vi "Rhythm-Initialize.vi"(0 "Rhythm":T2={"Method"=enum."Telegraph", "Waveform"=enum."Click", "Time"={"Ramp (ms)"=1.0, "Duration (ms)"=2.0, "Interval (ms)"=1.0}, "Expr"="", "Pattern"={"# rand"=0.0, "reg fraction"=0.0, "Rcyc"=0, "pattern"=enum."RAND-REG", "Lsignal (cyc)"={"Min"=0, "Max"=0}, "Trans (cyc)"={"Min"=0, "Max"=0}}} caption="ToneCloud", 7 "Sampling rate (Hz)":dbl=50000.0, 9 "Npts":i32, 11 "error in (no error)":errorcluster) -> (3 "#frames":i32, 4 "Values":dbl[](array[numeric]), 6 "Mask":i32[](array[numeric]), 8 "Data":T1, 15 "error out":errorcluster)   [LabVIEW 2020]
uses:
  Rhythm-Properties.ctl
  Rhythm-Data.ctl
  Rhythm-Initialization Action.ctl
  Utility VIs/Math VIs/LinSpace (x0-dx-npts).vi
  Utility VIs/Array Manipulation VIs/Irregular Array Subset (I32).vi
  <vilib>/Analysis/1siggen.llb/Riffle Array (I32).vi
  <vilib>/Analysis/NI_AALBase.lvlib
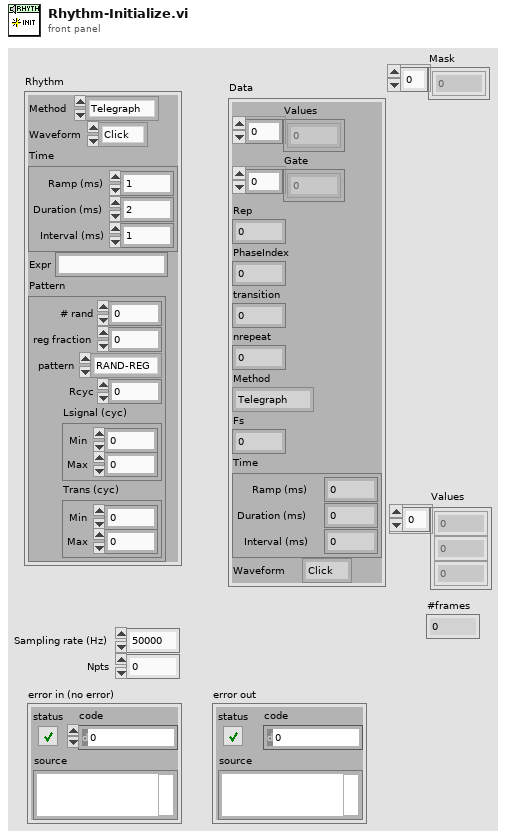
[diagram p1: front panel]
types:
  T1 = typedef "Rhythm-Data.ctl" = cluster{"Values":dbl[], "Gate":dbl[], "Rep":i32, "PhaseIndex":i32, "transition":i32, "nrepeat":i32, "Method":enum16{"Telegraph", "Interval"}, "Fs":dbl, "Time":cluster{"Ramp (ms)":dbl, "Duration (ms)":dbl, "Interval (ms)":dbl}, "Waveform":enum16{"Click", "Noise"}}
  T2 = typedef "Rhythm-Properties.ctl" = cluster{"Method":enum16{"Telegraph", "Interval"}, "Waveform":enum16{"Click", "Noise"}, "Time":cluster{"Ramp (ms)":dbl, "Duration (ms)":dbl, "Interval (ms)":dbl}, "Expr":string, "Pattern":cluster{"# rand":dbl, "reg fraction":dbl, "Rcyc":i32, "pattern":enum16{"RAND-REG", "REG-RAND", "RAND", "REG", "STEP", "CF"}, "Lsignal (cyc)":cluster{"Min":i32, "Max":i32}, "Trans (cyc)":cluster{"Min":i32, "Max":i32}}}
  T3 = typedef "Rhythm-Initialization Action.ctl" = enum16{"Start", "Rand", "Reg", "Titrate", "Signal", "Done"}
  T4 = cluster{"Duration (ms)":dbl, "Interval (ms)":dbl, "Ramp (ms)":dbl}
  T5 = cluster{"Ramp (ms)":dbl, "Duration (ms)":dbl, "Interval (ms)":dbl}
  T6 = enum16{"RAND-REG", "REG-RAND", "RAND", "REG", "STEP", "CF"}
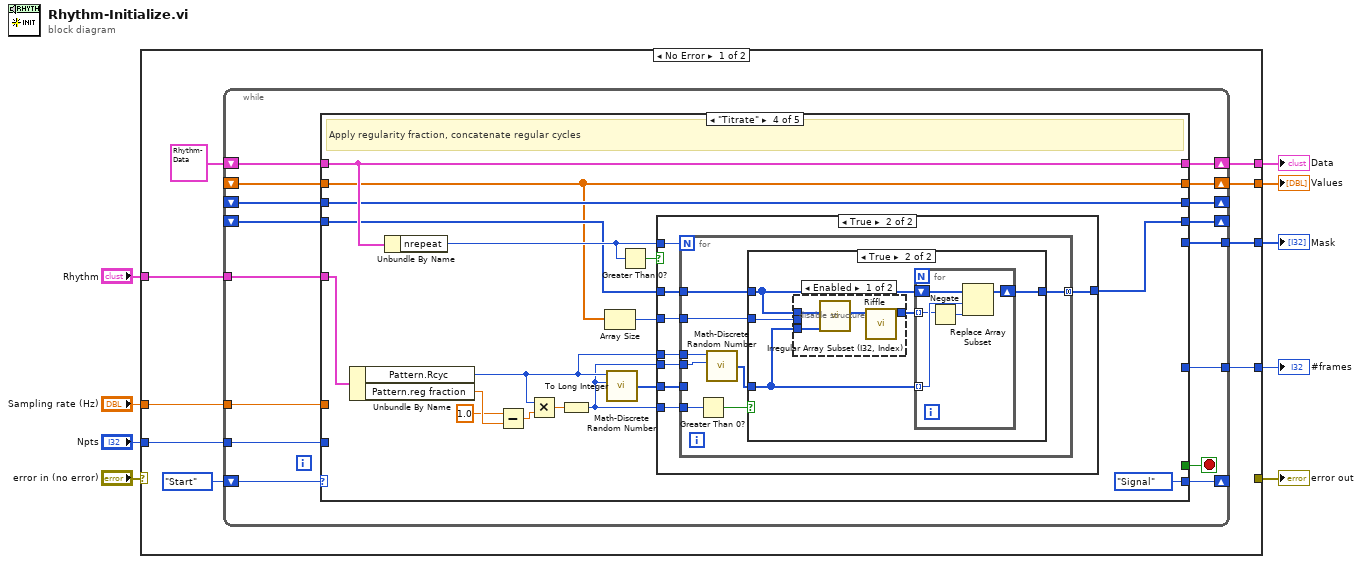
[diagram p0: block diagram]
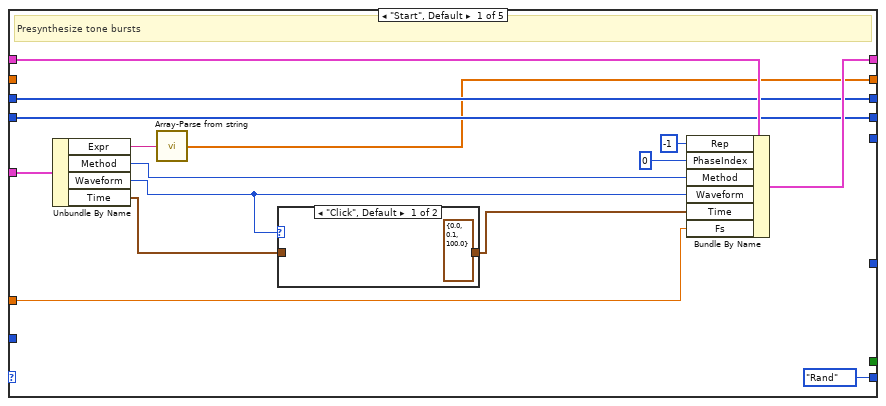
[diagram p2: hidden frame]
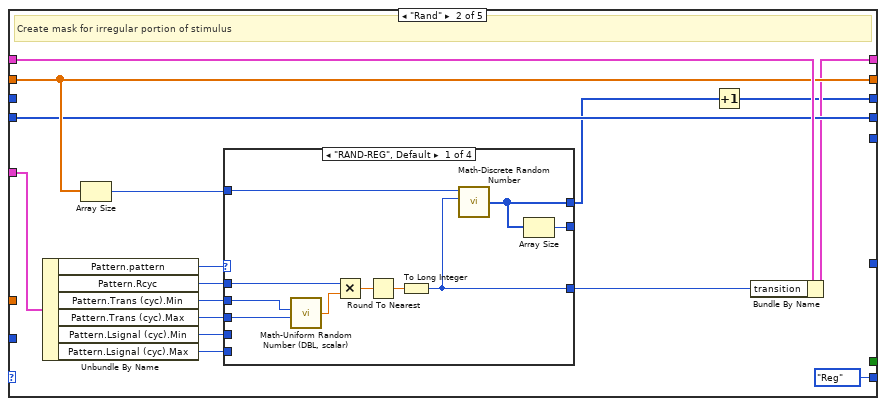
[diagram p4: hidden frame]
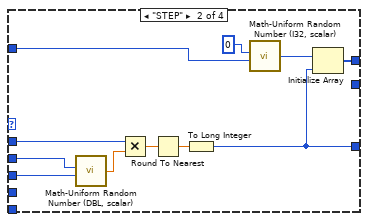
[diagram p5: hidden frame]
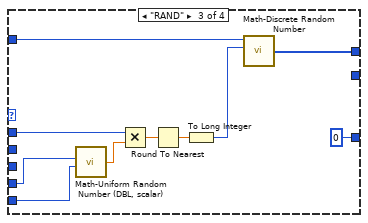
[diagram p6: hidden frame]
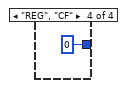
[diagram p7: hidden frame]
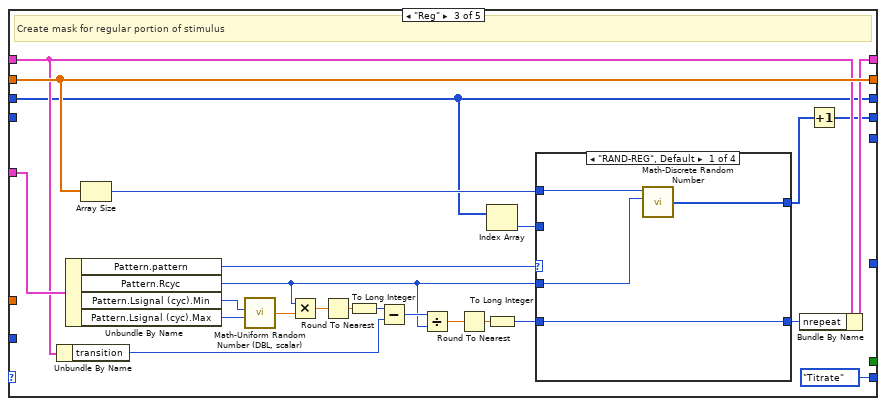
[diagram p8: hidden frame]
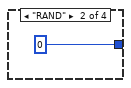
[diagram p9: hidden frame]
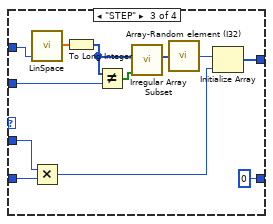
[diagram p10: hidden frame]
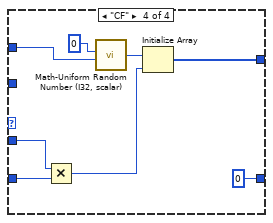
[diagram p11: hidden frame]
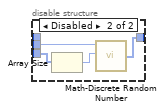
[diagram p14: hidden frame]
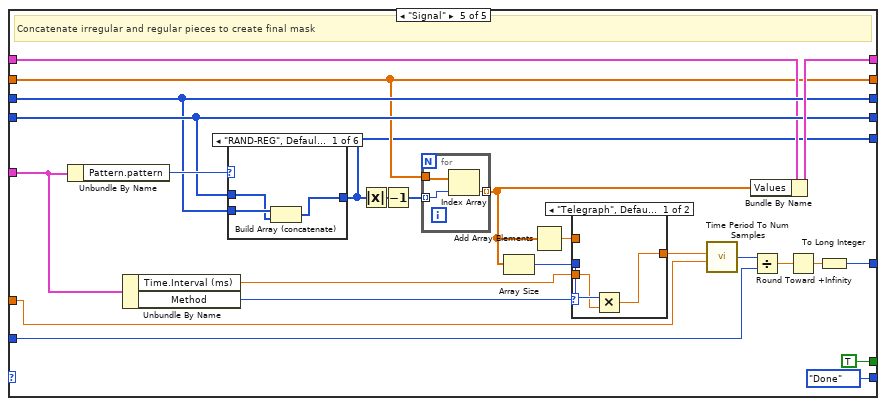
[diagram p15: hidden frame]
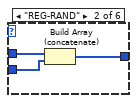
[diagram p17: hidden frame]
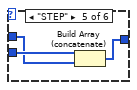
[diagram p20: hidden frame]
diagram:
  n1 = case shown="No Error" "error in (no error)" {
    selector: "error in (no error)" -> [_ w245]
    tunnel: [_ w245] -> w6
    tunnel: "Sampling rate (Hz)" -> [w17 _]
    tunnel: "Npts" -> [w13 _]
    tunnel: "Rhythm" -> [w16 _]
    tunnel: [w18 _] -> w4
    tunnel: [w14 _] -> w3
    tunnel: [w12 _] -> w2
    tunnel: [w10 _] -> w1
    frame No Error {
      n2 = while {
        tunnel: w17 -> [w33]
        tunnel: w16 -> [w32]
        shift-right: [w34] -> w18
        shift-left: T1 {"Values"=[], "Gate"=[], "Rep"=0, "PhaseIndex"=0, "transition"=0, "nrepeat"=0, "Method"=enum."Telegraph", "Fs"=0.0, "Time"={"Ramp (ms)"=0.0, "Duration (ms)"=0.0, "Interval (ms)"=0.0}, "Waveform"=enum."Click"} ("Data") -> [w31]
        shift-right: [w30] -> _
        shift-left: _ -> [w29]
        shift-right: [w28] -> w14
        shift-left: _ -> [w27]
        shift-right: [w26] -> _
        shift-left: _ -> [w25]
        tunnel: w13 -> [w23]
        tunnel: [w22] -> w12
        shift-right: [w20] -> _
        shift-left: Rhythm-Initialization_Action."Start" -> [w21]
        tunnel: [w19] -> w10
        stop <- w24 stop-if-true
        n3 = case shown="\"Titrate\"" w21 {
          tunnel: [w49 w59 w108 w165 w225] -> w34
          tunnel: w33 -> [w39 _ _ _ w208]
          tunnel: w32 -> [w48 w67 w123 w164 w214]
          tunnel: w31 -> [w47 w66 w114 w165 w220]
          tunnel: [w46 w52 w104 w162 w222] -> w30
          tunnel: w29 -> [w46 _ w104 w162 w222]
          tunnel: [w43 w65 w122 w153 w213] -> w28
          tunnel: w27 -> [_ w65 w122 w153 w213]
          tunnel: [w45 w64 w100 w160 w223] -> w26
          tunnel: w25 -> [w45 w64 _ w154 w223]
          tunnel: [_ _ _ _ TRUE] -> w24
          tunnel: w23 -> [_ _ _ _ w219]
          tunnel: [_ _ _ _ w216] -> w22
          tunnel: [Rhythm-Initialization_Action."Rand" Rhythm-Initialization_Action."Reg" Rhythm-Initialization_Action."Titrate" Rhythm-Initialization_Action."Signal" Rhythm-Initialization_Action."Done"] -> w20
          tunnel: [_ _ _ _ w202] -> w19
          frame "Start", Default {
            # "Presynthesize tone bursts"
            n4 = Unbundle By Name(w48) -> ("Expr"=w44:string, "Method"=w41:enum16{"Telegraph", "Interval"}, "Waveform"=w38:enum16{"Click", "Noise"}, "Time"=w37:T5)
            n5 = call "Array-Parse from string.vi"("String"=w44) -> ("Array"=w43:dbl[])  [unwired: 13 in, 1 out]
            n6 = case shown="\"Click\", Default" w38 {
              tunnel: w37 -> [_ w51]
              tunnel: [T4 {"Duration (ms)"=0.0, "Interval (ms)"=0.1, "Ramp (ms)"=100.0} ("Time") w51] -> w36
              frame "Click", Default {
              }
              frame "Noise" {
              }
            }
            n7 = Bundle By Name(cluster=w47, "Rep"=-1, "PhaseIndex"=0 ("Index"), "Method"=w41, "Waveform"=w38, "Time"=w36, "Fs"=w39) -> (w49:T1)
          }
          frame "Rand" {
            # "Create mask for irregular portion of stimulus"
            n8 = Unbundle By Name(w67) -> ("Pattern.pattern"=w57:T6, "Pattern.Rcyc"=w61:i32, "Pattern.Trans (cyc).Min"=w63:i32, "Pattern.Trans (cyc).Max"=w62:i32, "Pattern.Lsignal (cyc).Min"=w56:i32, "Pattern.Lsignal (cyc).Max"=w55:i32)
            n9 = Array Size(array=w65) -> (size(s)=w60:i32)
            n10 = case shown="\"RAND-REG\", Default" w57 {
              tunnel: w63 -> [w77 w88 _ _]
              tunnel: w62 -> [w76 w87 _ _]
              tunnel: w61 -> [w75 w86 w98 _]
              tunnel: w60 -> [w74 w82 w97 _]
              tunnel: [w69 w79 w96 _] -> w54
              tunnel: [w70 w78 0 0] -> w58
              tunnel: w56 -> [_ _ w91 _]
              tunnel: w55 -> [_ _ w90 _]
              tunnel: [w68 _ _ _] -> _
              frame "RAND-REG", Default {
                n11 = call "Math-Uniform Random Number (DBL, scalar).vi"("Ymax"=w76, "Ymin"=w77) -> ("Random Value"=w73:dbl)  [unwired: 4 in]
                n12 = Multiply(x=w75, y=w73) -> (x*y=w72:dbl)
                n13 = Round To Nearest(number=w72) -> (nearest integer value=w71:dbl)
                n14 = To Long Integer(number=w71) -> (32bit integer=w70:i32)
                n15 = call "Math-Discrete Random Number.vi"("N"=w70, "samples"=w74) -> ("Random Values"=w69:i32[])  [unwired: 4 in]
                n16 = Array Size(array=w69) -> (size(s)=w68:i32)
              }
              frame "STEP" {
                n17 = call "Math-Uniform Random Number (DBL, scalar).vi"("Ymax"=w87, "Ymin"=w88) -> ("Random Value"=w85:dbl)  [unwired: 4 in]
                n18 = Multiply(x=w86, y=w85) -> (x*y=w84:dbl)
                n19 = Round To Nearest(number=w84) -> (nearest integer value=w83:dbl)
                n20 = To Long Integer(number=w83) -> (32bit integer=w78:i32)
                n21 = call "Math-Uniform Random Number (I32, scalar).vi"("Ymax"=w82, "Ymin"=0) -> ("Random Int"=w80:i32)  [unwired: 4 in]
                n22 = Initialize Array(w80, w78) -> (w79:i32[])
              }
              frame "RAND" {
                n23 = call "Math-Uniform Random Number (DBL, scalar).vi"("Ymax"=w90, "Ymin"=w91) -> ("Random Value"=w95:dbl)  [unwired: 4 in]
                n24 = Multiply(x=w98, y=w95) -> (x*y=w94:dbl)
                n25 = Round To Nearest(number=w94) -> (nearest integer value=w93:dbl)
                n26 = To Long Integer(number=w93) -> (32bit integer=w92:i32)
                n27 = call "Math-Discrete Random Number.vi"("N"=w92, "samples"=w97) -> ("Random Values"=w96:i32[])  [unwired: 4 in]
              }
              frame "REG", "CF" {
              }
            }
            n28 = Increment(x=w54) -> (x+1=w52:i32[])
            n29 = Bundle By Name(cluster=w66, "transition"=w58) -> (w59:T1)
          }
          frame "Reg" {
            # "Create mask for regular portion of stimulus"
            n30 = Unbundle By Name(w114) -> ("transition"=w112:i32)
            n31 = Unbundle By Name(w123) -> ("Pattern.pattern"=w106:T6, "Pattern.Rcyc"=w105:i32, "Pattern.Lsignal (cyc).Min"=w116:i32, "Pattern.Lsignal (cyc).Max"=w115:i32)
            n32 = Array Size(array=w122) -> (size(s)=w121:i32)
            n33 = call "Math-Uniform Random Number (DBL, scalar).vi"("Ymax"=w115, "Ymin"=w116) -> ("Random Value"=w117:dbl)  [unwired: 4 in]
            n34 = Multiply(x=w105, y=w117) -> (x*y=w118:dbl)
            n35 = Round To Nearest(number=w118) -> (nearest integer value=w119:dbl)
            n36 = To Long Integer(number=w119) -> (32bit integer=w113:i32)
            n37 = Subtract(x=w113, y=w112) -> (x-y=w111:i32)
            n38 = Divide(x=w111, y=w105) -> (x/y=w110:dbl)
            n39 = Round To Nearest(number=w110) -> (nearest integer value=w109:dbl)
            n40 = Index Array(array=w104) -> (element=w103:i32)  [unwired: 1 in]
            n41 = To Long Integer(number=w109) -> (32bit integer=w101:i32)
            n42 = case shown="\"RAND-REG\", Default" w106 {
              tunnel: w121 -> [w127 _ w133 w145]
              tunnel: [w126 _ w135 w141] -> w120
              tunnel: [w124 0 0 0] -> w107
              tunnel: w101 -> [w124 _ w138 w144]
              tunnel: w105 -> [w125 _ w137 w143]
              tunnel: w103 -> [_ _ w140 _]
              frame "RAND-REG", Default {
                n43 = call "Math-Discrete Random Number.vi"("N"=w125, "samples"=w127) -> ("Random Values"=w126:i32[])  [unwired: 4 in]
              }
              frame "RAND" {
              }
              frame "STEP" {
                n44 = call-poly "LinSpace.vi"("npts"=w133) -> ("Array"=w132:dbl[])  [unwired: 3 in, 1 out]
                n45 = Multiply(x=w137, y=w138) -> (x*y=w136:i32)
                n46 = To Long Integer(number=w132) -> (32bit integer=w130:i32[])
                n47 = Not Equal?(x=w130, y=w140) -> (x != y?=w131:bool[])
                n48 = call-poly "Irregular Array Subset.vi"("Mask"=w131, "Array"=w130) -> ("Array Subset"=w129:i32[])  [unwired: 8 in, 1 out]
                n49 = call "Array-Random element (I32).vi"("Array"=w129) -> ("Element"=w134:i32)  [unwired: 1 in, 1 out]
                n50 = Initialize Array(w134, w136) -> (w135:i32[])
              }
              frame "CF" {
                n51 = Multiply(x=w143, y=w144) -> (x*y=w142:i32)
                n52 = call "Math-Uniform Random Number (I32, scalar).vi"("Ymax"=w145, "Ymin"=0) -> ("Random Int"=w146:i32)  [unwired: 4 in]
                n53 = Initialize Array(w146, w142) -> (w141:i32[])
              }
            }
            n54 = Bundle By Name(cluster=w114, "nrepeat"=w107) -> (w108:T1)
            n55 = Increment(x=w120) -> (x+1=w100:i32[])
          }
          frame "Titrate" {
            # "Apply regularity fraction, concatenate regular cycles"
            n56 = Unbundle By Name(w164) -> ("Pattern.Rcyc"=w151:i32, "Pattern.reg fraction"=w156:dbl)
            n57 = Unbundle By Name(w165) -> ("nrepeat"=w159:i32)
            n58 = Subtract(x=1.0, y=w156) -> (x-y=w157:dbl)
            n59 = Multiply(x=w151, y=w157) -> (x*y=w163:dbl)
            n60 = To Long Integer(number=w163) -> (32bit integer=w150:i32)
            n61 = Array Size(array=w153) -> (size(s)=w152:i32)
            n62 = call "Math-Discrete Random Number.vi"("N"=w150, "samples"=w151) -> ("Random Values"=w161:i32[])  [unwired: 4 in]
            n63 = Greater Than 0?(x=w159) -> (x > 0?=w158:bool)
            n64 = case shown="True" w158 {
              tunnel: w159 -> [_ w174]
              tunnel: w154 -> [w166 w173]
              tunnel: w161 -> [_ w172]
              tunnel: w150 -> [_ w171]
              tunnel: [w166 w170] -> w160
              tunnel: w152 -> [_ w169]
              tunnel: w151 -> [_ w168]
              tunnel: w150 -> [_ w167]
              frame False {
              }
              frame True {
                n65 = for {
                  N: w174 -> [_]
                  tunnel: w173 -> [w180]
                  tunnel: w172 -> [_]
                  tunnel: w171 -> [w182]
                  tunnel: [w179] -> w170 mode=concatenating
                  tunnel: w169 -> [w178]
                  tunnel: w168 -> [w177]
                  tunnel: w167 -> [w176]
                  n66 = Greater Than 0?(x=w182) -> (x > 0?=w181:bool)
                  n67 = call "Math-Discrete Random Number.vi"("N"=w176, "samples"=w177) -> ("Random Values"=w175:i32[])  [unwired: 4 in]
                  n68 = case shown="True" w181 {
                    tunnel: w180 -> [w183 w188]
                    tunnel: w175 -> [_ w185]
                    tunnel: [w183 w187] -> w179
                    tunnel: w178 -> [_ w184]
                    frame False {
                    }
                    frame True {
                      n69 = disable-structure shown="Enabled" {
                        disable-tunnel: w188 -> [w191 _]
                        disable-tunnel: [w190 w193] -> w186
                        disable-tunnel: w185 -> [w189 w196]
                        disable-tunnel: w184 -> [_ w195]
                        frame Enabled {
                          n70 = call "Irregular Array Subset (I32, Index).vi"("Indices"=w189, "Array"=w191) -> ("Array Subset"=w192:i32[])  [unwired: 8 in, 1 out]
                          n71 = call-poly <vilib>:"Riffle.vi"("X"=w192) -> ("Riffled {X}"=w190:i32[])  [unwired: 8 in, 2 out]
                        }
                        frame Disabled {
                          n72 = Array Size(array=w196) -> (size(s)=w194:i32)
                          n73 = call "Math-Discrete Random Number.vi"("N"=w194, "samples"=w195) -> ("Random Values"=w193:i32[])  [unwired: 4 in]
                        }
                      }
                      n74 = for {
                        shift-right: [w200] -> w187
                        shift-left: w188 -> [w201]
                        tunnel: w186 -> [w198] mode=indexing
                        tunnel: w185 -> [w199] mode=indexing
                        n75 = Negate(x=w198) -> (-x=w197:i32)
                        n76 = Replace Array Subset(array=w201, new element=w197, index=w199) -> (w200:i32[])
                      }
                    }
                  }
                }
              }
            }
          }
          frame "Signal" {
            # "Concatenate irregular and regular pieces to create final mask"
            n77 = Unbundle By Name(w214) -> ("Pattern.pattern"=w224:T6)
            n78 = Unbundle By Name(w214) -> ("Time.Interval (ms)"=w205:dbl, "Method"=w212:enum16{"Telegraph", "Interval"})
            n79 = case shown="\"RAND-REG\", Default" w224 {
              tunnel: w223 -> [w234 w238 _ w240 w242 _]
              tunnel: w222 -> [w235 w237 w239 _ w243 w244]
              tunnel: [w233 w236 w239 w240 w241 w244] -> w202
              frame "RAND-REG", Default {
                n80 = Build Array (concatenate)(w235, w234) -> (w233:i32[])
              }
              frame "REG-RAND" {
                n81 = Build Array (concatenate)(w238, w237) -> (w236:i32[])
              }
              frame "RAND" {
              }
              frame "REG" {
              }
              frame "STEP" {
                n82 = Build Array (concatenate)(w243, w242) -> (w241:i32[])
              }
              frame "CF" {
              }
            }
            n83 = Absolute Value(x=w202) -> (abs(x)=w204:i32[])
            n84 = Decrement(x=w204) -> (x-1=w203:i32[])
            n85 = for {
              tunnel: w213 -> [w232]
              tunnel: w203 -> [w231] mode=indexing
              tunnel: [w230] -> w206 mode=indexing
              n86 = Index Array(array=w232, index=w231) -> (element=w230:dbl)
            }
            n87 = Array Size(array=w206) -> (size(s)=w207:i32)
            n88 = Add Array Elements(numeric array=w206) -> (sum=w211:dbl)
            n89 = case shown="\"Telegraph\", Default" w212 {
              tunnel: w207 -> [w228 _]
              tunnel: w205 -> [w227 _]
              tunnel: [w226 w229] -> w209
              tunnel: w211 -> [_ w229]
              frame "Telegraph", Default {
                n90 = Multiply(x=w228, y=w227) -> (x*y=w226:dbl)
              }
              frame "Interval" {
              }
            }
            n91 = call "Time Period To Num Samples.vi"("Duration (ms)"=w209, "Sampling rate (Hz)"=w208) -> ("Samples"=w210:i32)  [unwired: 5 in]
            n92 = Bundle By Name(cluster=w220, "Values"=w206) -> (w225:T1)
            n93 = Divide(x=w210, y=w219) -> (x/y=w218:dbl)
            n94 = Round Toward +Infinity(x=w218) -> (ceil(x): smallest int >= x=w217:dbl)
            n95 = To Long Integer(number=w217) -> (32bit integer=w216:i32)
          }
        }
      }
    }
    frame Error {
    }
  }
  "error out" <- w6
  "Data" <- w4
  "Values" <- w3
  "#frames" <- w2
  "Mask" <- w1
